vi "Copy To IMAQ.vi"() -> ()   [LabVIEW 2020]
uses:
  g_ar_toolkit.image/Image Size (Fixed).ctl
  g_ar_toolkit.image/Raw Memory Information.ctl
  g_ar_toolkit.image/Raw Memory Information Dimension.ctl
  g_ar_toolkit.image/DrawImageARGB.vi
  g_ar_toolkit.image/CreateEmptyImageARGB.vi/3321fa97-f432-4e1e-8db9-a0df79aed21b.vi
  g_ar_toolkit.image/DrawImageARGB.vi/8cd07b1b-062e-4fe4-9e87-2eb3dc89fe0e.vi
  g_ar_toolkit.image/CopyImageToRawMemoryARGB.vi/01eda17f-9221-4e43-bf47-cf9d986167a3.vi
  g_ar_toolkit.image/ARGBColourToU32.vi
  <vilib>/Utility/error.llb/Error Cluster From Error Code.vi
  <vilib>/vision/EDVR.llb/IMAQ ImageToEDVR 2D U32.vi
  g_ar_toolkit.image/g_ar_toolkit.image.lvlib
panel:
  in  "Mode":T1(ring)
  out "IMAQ":T2(plugin-control)
  out "Input":picture
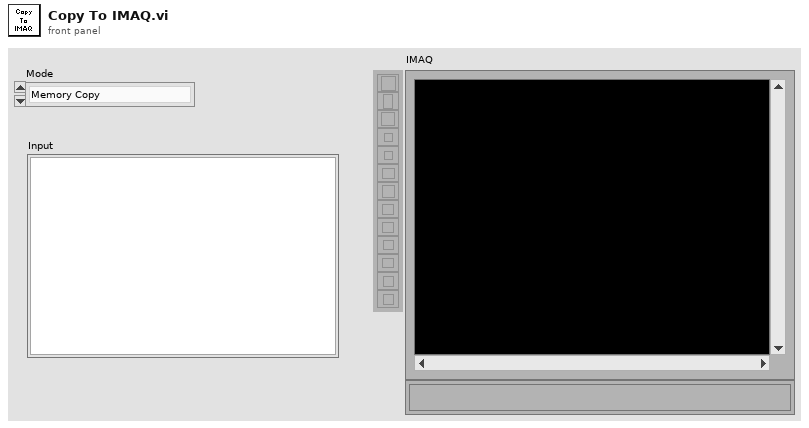
[diagram p1: front panel]
types:
  T1 = enum16{"Memory Copy", "EDVR Access", "Array Values"}
  T2 = typedef "IMAQ Image.ctl" = refnum<image>
  T3 = typedef "g_ar_toolkit.image.lvlib/Image Size (Fixed).ctl" = cluster{"Width":u16, "Height":u16}
  T4 = typedef "Image Type" = u32
  T5 = enum32{"Map Pixel Pointer", "Unmap Pixel Pointer", "Get Pixels Infos"}
  T6 = typedef "g_ar_toolkit.image.lvlib/Raw Memory Information.ctl" = cluster{"Memory Address":u64, "Dimension 0":T7, "Dimension 1":T7}
  T7 = typedef "g_ar_toolkit.image.lvlib/Raw Memory Information Dimension.ctl" = cluster{"Size":u16, "Stride":u32}
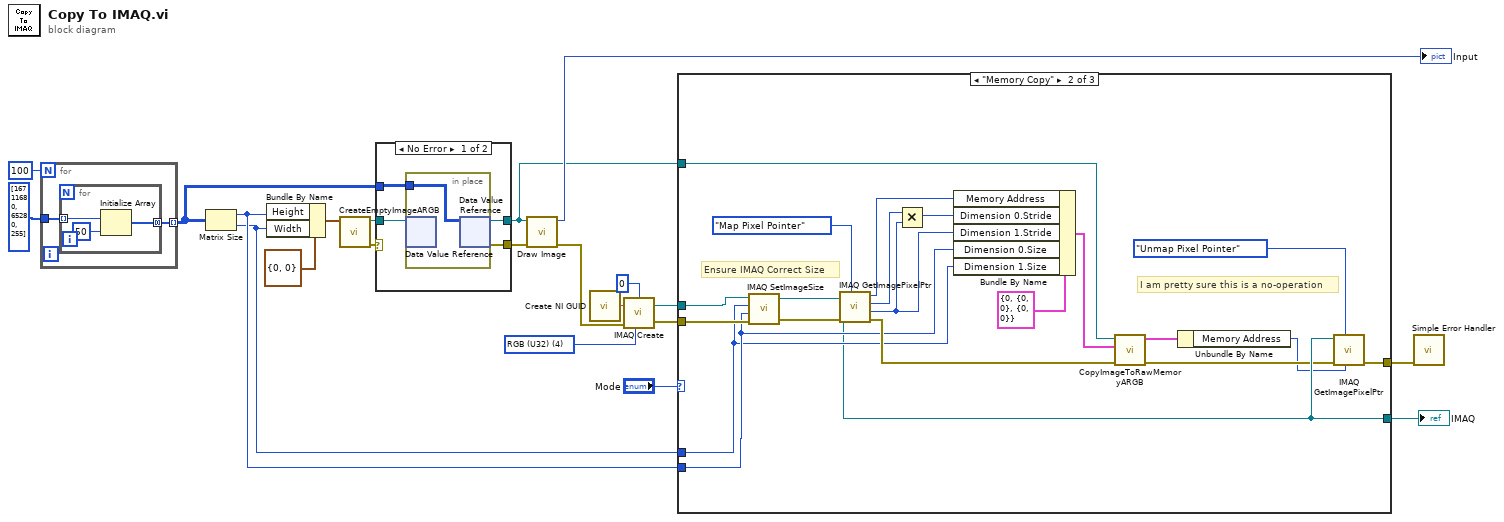
[diagram p0: block diagram]
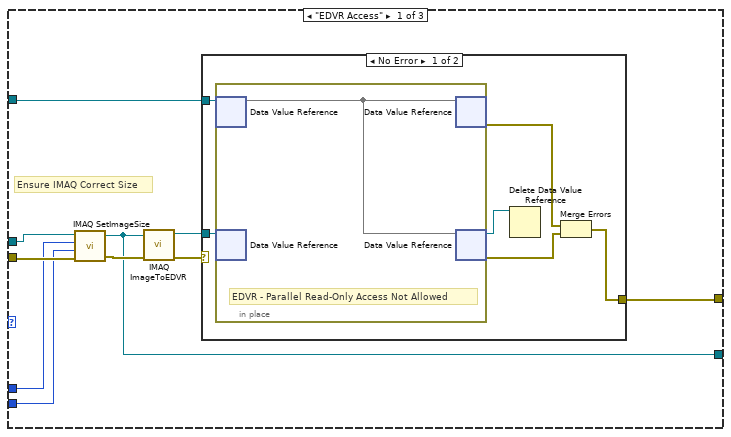
[diagram p3: hidden frame]
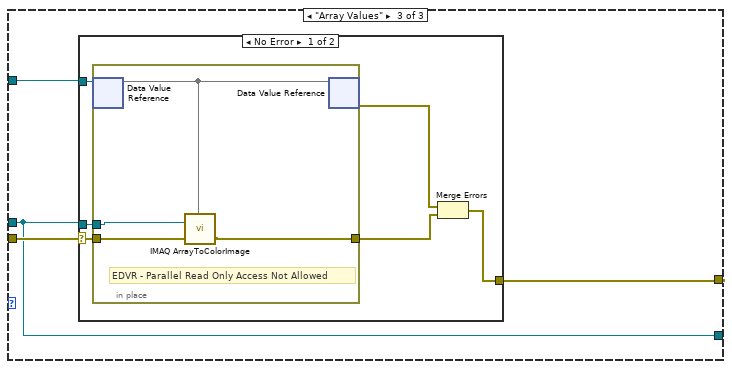
[diagram p5: hidden frame]
diagram:
  w19 = T4 4 items=["Grayscale (U8)", "Grayscale (I16)", "Grayscale (SGL)", "Complex (CSG)", "RGB (U32)", "HSL (U32)", "RGB (U64)", "Grayscale (U16)"] ("Image Type")
  n1 = for {
    N: 100 -> [_]
    tunnel: u32[] [16711680, 65280, 255] ("color(black)") -> [w23]
    tunnel: [w22] -> w5 mode=indexing
    n2 = for {
      tunnel: w23 -> [w26] mode=indexing
      tunnel: [w24] -> w22 mode=concatenating
      n3 = Initialize Array(w26, 50 ("dimension size")) -> (w24:u32[])
    }
  }
  n4 = Matrix Size(0:w5) -> (1:w13:i32, 2:w12:i32)
  n5 = Bundle By Name(cluster=T3 {"Width"=0, "Height"=0} ("Preallocated Image Size (Default: 0,0)"), "Height"=w13, "Width"=w12) -> (w16:T3)
  n6 = call "CreateEmptyImageARGB.vi"("Preallocated Image Size (Default: 0,0)"=w16) -> ("error out"=w2:errorcluster, "New ARGB Image"=w6:refnum<data-value>)  [unwired: 9 in]
  n7 = case shown="No Error" w2 {
    selector: w2 -> [_ w33]
    tunnel: w6 -> [w30 w32]
    tunnel: w5 -> [w29 _]
    tunnel: [w28 w33] -> w4
    tunnel: [w27 w32] -> w3
    frame No Error {
      n8 = in-place {
        in-place-border: w29 -> [w31]
        n9 = in-place-dvr #1(w30) -> ()  [unwired: 2 out]
        n10 = in-place-dvr #1(w31) -> (w27:refnum<data-value>, w28:errorcluster)
      }
    }
    frame Error {
    }
  }
  n11 = call-poly "Draw Image.vi"("error in (no error)"=w4, "ARGB Image Source"=w3) -> ("error out"=w11:errorcluster, "Picture"=→"Input":picture)  [unwired: 8 in]
  n12 = call <vilib>:"Create NI GUID.vi"() -> ("NI GUID"=w7:string)
  n13 = call "IMAQ Create"("Border Size"=0, "Image Name"=w7, "Image Type"=w19, "error in (no error)"=w11) -> ("New Image"=w14:T2, "error out"=w15:errorcluster)  [unwired: 1 in]
  n14 = case shown="\"Memory Copy\"" "Mode" {
    tunnel: w15 -> [w40 w70 w75]
    tunnel: w14 -> [w39 w69 w72]
    tunnel: w13 -> [w35 w68 _]
    tunnel: w12 -> [w34 w67 _]
    tunnel: [w37 w66 w72] -> w9
    tunnel: [w38 w65 w73] -> w8
    tunnel: w3 -> [w36 w64 w74]
    frame "EDVR Access" {
      # "Ensure IMAQ Correct Size"
      n15 = call "IMAQ SetImageSize"("error in (no error)"=w40, "Y Resolution"=w35, "X Resolution"=w34, "Image"=w39) -> ("error out"=w43:errorcluster, "Image Out"=w37:T2)  [unwired: 1 in]
      n16 = call-poly <vilib>:"IMAQ ImageToEDVR.vi"("error out"=w43, "Image"=w37) -> ("error out"=w41:errorcluster, "EDVR 2D U32"=w42:refnum<data-value>)  [unwired: 7 in, 1 out]
      n17 = case shown="No Error" w41 {
        selector: w41 -> [_ w51]
        tunnel: w42 -> [w49 _]
        tunnel: [w45 w51] -> w38
        tunnel: w36 -> [w44 _]
        frame No Error {
          n18 = in-place {
            # "EDVR - Parallel Read-Only Access Not Allowed"
            n19 = in-place-dvr #2(w44) -> (w50:u32[][])  [unwired: 1 out]
            n20 = in-place-dvr #3(w49) -> ()  [unwired: 2 out]
            n21 = in-place-dvr #2(w50) -> (w47:errorcluster)  [unwired: 1 out]
            n22 = in-place-dvr #3(w50) -> (w48:refnum<data-value>, w46:errorcluster)
          }
          n23 = Delete Data Value Reference(data value reference=w48) -> ()  [unwired: 1 in, 2 out]
          n24 = Merge Errors(w47, w46) -> (w45:errorcluster)
        }
        frame Error {
        }
      }
    }
    frame "Memory Copy" {
      # "Ensure IMAQ Correct Size"
      # "I am pretty sure this is a no-operation"
      n25 = call "IMAQ SetImageSize"("error in (no error)"=w70, "Y Resolution"=w68, "X Resolution"=w67, "Image"=w69) -> ("error out"=w58:errorcluster, "Image Out"=w66:T2)  [unwired: 1 in]
      n26 = call "IMAQ GetImagePixelPtr"("Function"=T5."Map Pixel Pointer", "error in (no error)"=w58, "Image"=w66) -> ("error out"=w71:errorcluster, "Pixel Size (Bytes)"=w52:i32, "LineWidth(Pixels)"=w60:i32, "Pixel Pointer out"=w63:u64)  [unwired: 3 in, 2 out]
      n27 = Multiply(x=w60, y=w52) -> (x*y=w53:i32)
      n28 = Bundle By Name(cluster=T6 {"Memory Address"=0, "Dimension 0"={"Size"=0, "Stride"=0}, "Dimension 1"={"Size"=0, "Stride"=0}} ("Source"), "Memory Address"=w63, "Dimension 0.Stride"=w53, "Dimension 1.Stride"=w52, "Dimension 0.Size"=w68, "Dimension 1.Size"=w67) -> (w57:T6)
      n29 = call "CopyImageToRawMemoryARGB.vi"("error in (no error)"=w71, "Destination"=w57, "ARGB Image Source"=w64) -> ("error out"=w56:errorcluster, "Destination (Duplcate)"=w55:T6)  [unwired: 7 in]
      n30 = Unbundle By Name(w55) -> ("Memory Address"=w54:u64)
      n31 = call "IMAQ GetImagePixelPtr"("Pixel Pointer in"=w54, "Function"=T5."Unmap Pixel Pointer", "error in (no error)"=w56, "Image"=w66) -> ("error out"=w65:errorcluster)  [unwired: 2 in, 5 out]
    }
    frame "Array Values" {
      n32 = case shown="No Error" w75 {
        selector: w75 -> [w77 w86]
        tunnel: w74 -> [w81 _]
        tunnel: [w79 w86] -> w73
        tunnel: w72 -> [w78 _]
        frame No Error {
          n33 = in-place {
            in-place-border: w78 -> [w85]
            in-place-border: w77 -> [w84]
            in-place-border: [w82] -> w76
            # "EDVR - Parallel Read Only Access Not Allowed"
            n34 = in-place-dvr #4(w81) -> (w83:u32[][])  [unwired: 1 out]
            n35 = call "IMAQ ArrayToColorImage"("Image Pixels (U32)"=w83, "Image"=w85, "error in (no error)"=w84) -> ("error out"=w82:errorcluster)  [unwired: 2 in, 1 out]
            n36 = in-place-dvr #4(w83) -> (w80:errorcluster)  [unwired: 1 out]
          }
          n37 = Merge Errors(w80, w76) -> (w79:errorcluster)
        }
        frame Error {
        }
      }
    }
  }
  "IMAQ" <- w9
  n38 = call <vilib>:"Simple Error Handler.vi"("error in (no error)"=w8) -> ()  [unwired: 4 in, 5 out]
